vi "getLastFile (SubVI).vi"(9 "Datafile (1=last)":i32, 10 "pattern":string, 11 "Session path":path) -> (3 "path out":path)   [LabVIEW 2014]
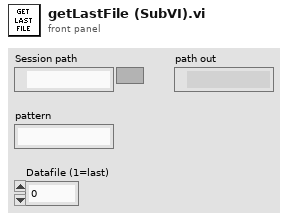
[diagram p1: front panel]
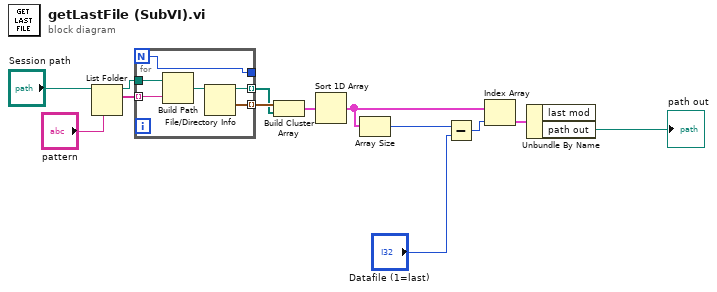
[diagram p0: block diagram]
diagram:
  n1 = List Folder(path="Session path", pattern="pattern") -> (path out=w2:path, filenames=w1:string[])  [unwired: 2 in, 2 out]
  n2 = for {
    N -> [w14]
    tunnel: w1 -> [w19] mode=indexing
    tunnel: w2 -> [w18]
    tunnel: [w16] -> w5 mode=indexing
    tunnel: [w15] -> w4 mode=indexing
    tunnel: [w14] -> _
    n3 = Build Path(base path=w18, name or relative path=w19) -> (appended path=w17:path)
    n4 = File/Directory Info(path=w17) -> (path out=w15:path, last mod=w16:timestamp)  [unwired: 1 in, 5 out]
  }
  n5 = Build Cluster Array(w5, w4) -> (w6:cluster{"last mod":timestamp, "path out":path}[])
  n6 = Sort 1D Array(array=w6) -> (sorted array=w10:cluster{"last mod":timestamp, "path out":path}[])
  n7 = Array Size(array=w10) -> (size(s)=w11:i32)
  n8 = Subtract(x=w11, y="Datafile (1=last)") -> (x-y=w12:i32)
  n9 = Index Array(array=w10, index=w12) -> (element=w8:cluster{"last mod":timestamp, "path out":path})
  n10 = Unbundle By Name(w8) -> ("path out"=→"path out":path)  [unwired: 1 out]
